vi "gather 2d info vision.vi"(6 "channel 0-4 energy in":u32[][](array[numeric]), 8 "error in (no error)":errorcluster, 10 "which gate":u16(ring) items=["pulser", "gate 1", "gate 2", "gate 3", "none"], 11 "New Image":i32[][](array[numeric])) -> (0 "Y name output":string, 1 "X name output":string, 2 "sum of counts out":i32, 3 "New Image out":i32[][](array[numeric]), 4 "Peak height out":i32[][](array[numeric]), 7 "2d width":i32[](array[numeric]), 9 "error out":errorcluster)   [LabVIEW 2016]
doc: "This takes all of the values exported from the pixie and determines if it\nfits within a defined region"
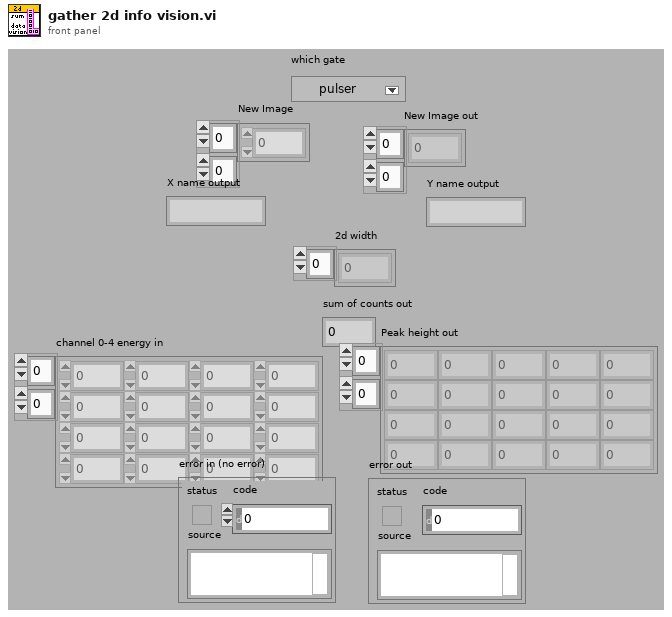
[diagram p1: front panel]
types:
  T1 = typedef "energy 2d selection.ctl" = string
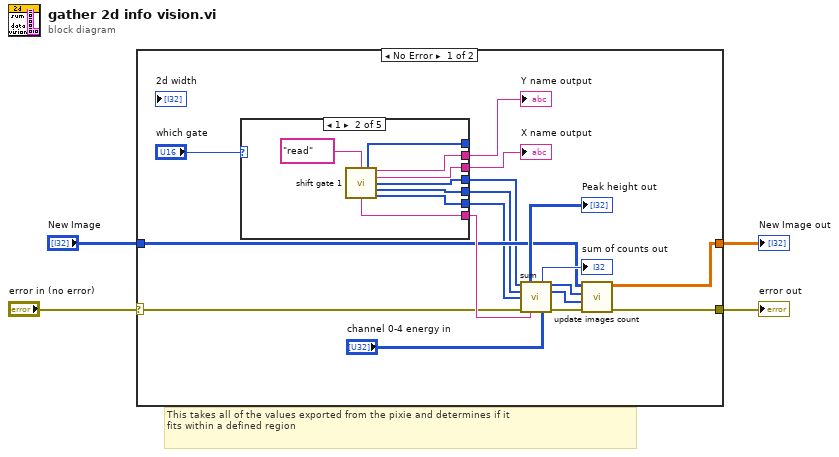
[diagram p0: block diagram]
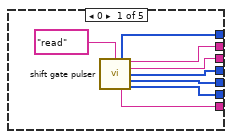
[diagram p2: hidden frame]
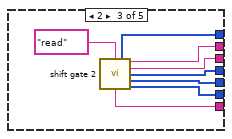
[diagram p3: hidden frame]
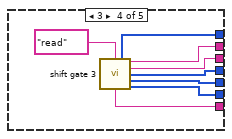
[diagram p4: hidden frame]
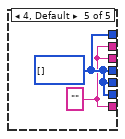
[diagram p5: hidden frame]
diagram:
  # "This takes all of the values exported from the pixie and determines if it\nfits within a defined region"
  n1 = case shown="No Error" "error in (no error)" {
    selector: "error in (no error)" -> [w8 w56]
    tunnel: "New Image" -> [w15 w57]
    tunnel: [w14 w57] -> w3
    tunnel: [w13 w56] -> w2
    frame No Error {
      n2 = case shown="1" "which gate" {
        tunnel: [w29 w37 w45 w53 w54] -> w16
        tunnel: [w28 w36 w38 w46 w54] -> w18
        tunnel: [w27 w35 w44 w52 w54] -> w17
        tunnel: [w26 w34 w43 w51 w55] -> w11
        tunnel: [w25 w33 w42 w50 w55] -> w12
        tunnel: [w24 w32 w41 w49 w55] -> w9
        tunnel: [w22 w30 w39 w47 w55] -> _
        frame 0 {
          n3 = call "shift gate pulser.vi"("shift control"="read") -> ("2d array width output"=w22:i32[], "X name output"=w27:string, "Y name  output"=w29:string, "X range output"=w24:i32[], "Y range Max output"=w25:i32[], "Energy 2d gate out"=w28:T1, "Y range Min output"=w26:i32[])  [unwired: 8 in]
        }
        frame 1 {
          n4 = call "shift gate 1.vi"("shift control"="read") -> ("2d  array width output"=w30:i32[], "X name output"=w35:string, "Y name  output"=w37:string, "X range output"=w32:i32[], "Y range Max output"=w33:i32[], "Energy 2d gate out"=w36:T1, "Y range Min output"=w34:i32[])  [unwired: 8 in]
        }
        frame 2 {
          n5 = call "shift gate 2.vi"("shift control"="read") -> ("2d position array output"=w39:i32[], "X name output"=w44:string, "Y name  output"=w45:string, "X range output"=w41:i32[], "Y range Max output"=w42:i32[], "Energy 2d gate out"=w38:T1, "Y range Min output"=w43:i32[])  [unwired: 8 in]
        }
        frame 3 {
          n6 = call "shift gate 3.vi"("shift control"="read") -> ("2d location array output"=w47:i32[], "X name output"=w52:string, "Y name  output"=w53:string, "X range output"=w49:i32[], "Y range Max output"=w50:i32[], "Energy 2d gate out"=w46:T1, "Y range Min output"=w51:i32[])  [unwired: 8 in]
        }
        frame 4, Default {
          w55 = i32[] [] ("X range output")
          w54 = "" ("X name output")
        }
      }
      "Y name output" <- w17
      "X name output" <- w16
      n7 = call "sum.vi"("X range output"=w9, "Y range Max output"=w12, "Y range Min output"=w11, "error in (no error)"=w8, "Energy 2d gate out"=w18, "Peak height  in"="channel 0-4 energy in") -> ("Peak height out"=→"Peak height out":u16[][], "sum of counts out"=→"sum of counts out":i32, "X output array"=w6:u16[], "Y range  output"=w5:u16[], "error out"=w10:errorcluster)  [unwired: 5 in]
      n8 = call "update images count.vi"("error in (no error)"=w10, "Y axis data"=w5, "x axis data"=w6, "Image in"=w15) -> ("error out"=w13:errorcluster, "Image Out"=w14:dbl[][])  [unwired: 6 in]
    }
    frame Error {
    }
  }
  "New Image out" <- w3
  "error out" <- w2
